vi "Begin.vi"(8 "error in":errorcluster) -> (0 "error out":errorcluster)   [LabVIEW 2014]
doc: "Called before other user functions, this VI is expected to open initial I/O refnums, load in file data, and do all program initialization. Notice that the <B>error out</B> terminal is simply used for data flow. Wiring it to other structures or subVIs ensures that this VI runs first."
uses:
  <vilib>/Rock Robotics/WPI/DriverStation/WPI_DriverStationRobotMode2.ctl
  <vilib>/Rock Robotics/WPI/Joystick/WPI_JoystickDeviceEnum.ctl
  <vilib>/Rock Robotics/SystemInterfaces/DIO/FPGA_DIOChannel.ctl
  <vilib>/Rock Robotics/SystemInterfaces/spilib/spi_bus.ctl
  <vilib>/Rock Robotics/WPI/SafetyOutput/WPI_SafetyOutputConfigMenu.ctl
  <vilib>/Rock Robotics/SystemInterfaces/DIO/FPGA_DIOPWMChannel.ctl
  <vilib>/Rock Robotics/SystemInterfaces/DIO/FPGA_DIORelayChannel.ctl
  <vilib>/Rock Robotics/WPI/Relay/WPI_RelayValue.ctl
  <vilib>/Rock Robotics/SystemInterfaces/i2clib/i2c_bus.ctl
  Robot Global Data.vi
  <vilib>/Rock Robotics/WPI/Counter/WPI_CounterDigitalInputToDigitalSource.vi
  <vilib>/Rock Robotics/WPI/Switch/WPI_SwitchOpenLimit.vi
  <vilib>/Rock Robotics/WPI/RobotDrive/WPI_RobotDriveOpen4MotorWithTalon.vi
  <vilib>/Rock Robotics/WPI/RobotDrive/WPI_RobotDriveOpen4MotorWithCANTalonSRX.vi
  <vilib>/Rock Robotics/WPI/MotorControl/WPI_MotorControlOpen Talon.vi
  SimpleGyro/SimpleGyro.lvlib
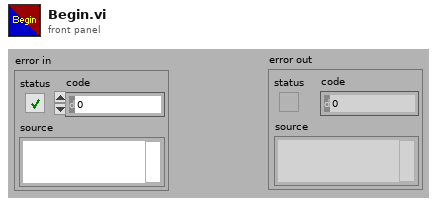
[diagram p1: front panel]
types:
  T1 = typedef "spi_bus.ctl" = enum16{"SPI On-Board, CS0", "SPI On-Board, CS1", "SPI On-Board, CS2", "SPI On-Board, CS3", "SPI MXP", "Invalid"}
  T2 = typedef "FPGA_DIOChannel.ctl" = enum8{"DIO 0", "DIO 1", "DIO 2", "DIO 3", "DIO 4", "DIO 5", "DIO 6", "DIO 7", "DIO 8", "DIO 9", "DIO MXP 0", "DIO MXP 1", "DIO MXP 2", "DIO MXP 3", "DIO MXP 4", "DIO MXP 5", "DIO MXP 6", "DIO MXP 7", "DIO MXP 8", "DIO MXP 9", "DIO MXP 10", "DIO MXP 11", "DIO MXP 12", "DIO MXP 13", "DIO MXP 14", "DIO MXP 15", "Invalid"}
  T3 = typedef "WPI_JoystickDeviceEnum.ctl" = enum16{"USB 0", "USB 1", "USB 2", "USB 3", "USB 4", "USB 5"}
  T4 = typedef "WPI_DriverStationRobotMode2.ctl" = enum16{"Autonomous Disabled", "Autonomous Enabled", "Teleop Disabled", "Teleop Enabled", "Disconnected", "Finish", "Test Disabled", "Test Enabled", "Emergency Stopped"}
  T5 = typedef "WPI_SafetyOutputConfigMenu.ctl" = enum16{"Enable", "Disable"}
  T6 = typedef "FPGA_DIORelayChannel.ctl" = enum8{"Relay 0", "Relay 1", "Relay 2", "Relay 3", "Invalid"}
  T7 = typedef "FPGA_DIOPWMChannel.ctl" = enum8{"PWM 0", "PWM 1", "PWM 2", "PWM 3", "PWM 4", "PWM 5", "PWM 6", "PWM 7", "PWM 8", "PWM 9", "PWM MXP 0", "PWM MXP 1", "PWM MXP 2", "PWM MXP 3", "PWM MXP 4", "PWM MXP 5", "PWM MXP 6", "PWM MXP 7", "PWM MXP 8", "PWM MXP 9", "Invalid"}
  T8 = typedef "WPI_RobotDriveDevRef.ctl" = cluster{"DevStatus":errorcluster, "Motors[]":T9[], "Square Inputs":bool, "Max Output":dbl}
  T9 = typedef "WPI_MotorControlDeviceRef.ctl" = cluster{"DeviceStatus":errorcluster, "Type":T10, "PWM":cluster{"Controller":T11, "PWM Channel":T7, "DeadBand":T12}, "CAN":cluster{"Device Number":u8, "Control Mode":T13, "Semaphore":T14, "Max Vout":dbl, "TalonSRX Control Mode":T15}, "Invert":bool, "TransformRef":T16, "InvTransformRef":T16}
  T10 = typedef "WPI_MotorControlType.ctl" = enum16{"PWM", "CAN", "CANTalonSRX"}
  T11 = typedef "FPGA_TypedefDigitalModule.ctl" = enum16{"Controller 1"}
  T12 = typedef "WPI_PWMDeadband.ctl" = cluster{"Name":string, "maxPositivePwm":i32, "minPositivePwm":i32, "centerPwm":i32, "maxNegativePwm":i32, "minNegativePwm":i32, "angularRange":u16}
  T13 = typedef "WPI_CANJaguar_ControlMode.ctl" = enum8{"Percent VBus", "Current", "Speed", "Position", "Voltage"}
  T14 = typedef "Semaphore RefNum" = refnum<k1>
  T15 = typedef "WPI_CANTalonSRX_APIControlMode.ctl" = enum8{"Percent VBus", "Speed", "Position", "Slave", "Unchanged / Invalid"}
  T16 = typedef "WPI_PWMTransform_ConPane.ctl" = refnum<vi>
  T17 = typedef "WPI_DigitalInputDevRef.ctl" = cluster{"DevStatus":errorcluster, "DIO Channel":T2, "Controller":T11}
  T18 = typedef "FPGA_CounterEncoderSourceConvertionLVSourceType.ctl" = cluster{"DevStatus":errorcluster, "AnalogTriggerMode?":bool, "DigitalMode":cluster{"Controller":T11, "DIO Channel":T19}, "AnalogTriggerMode":cluster{"AnalogTriggerIndex":T20, "OutputType":T21}}
  T19 = typedef "FPGA_DIODigitalSourceChannel.ctl" = enum8{"DIO 0", "DIO 1", "DIO 2", "DIO 3", "DIO 4", "DIO 5", "DIO 6", "DIO 7", "DIO 8", "DIO 9", "DIO MXP 0", "DIO MXP 1", "DIO MXP 2", "DIO MXP 3", "DIO MXP 4", "DIO MXP 5", "DIO MXP 6", "DIO MXP 7", "DIO MXP 8", "DIO MXP 9", "DIO MXP 10", "DIO MXP 11", "DIO MXP 12", "DIO MXP 13", "DIO MXP 14", "DIO MXP 15", "Disabled"}
  T20 = typedef "FPGA_AnalogTriggerIndex.ctl" = enum8{"Trig 0", "Trig 1", "Trig 2", "Trig 3", "Trig 4", "Trig 5", "Trig 6", "Trig 7", "Invalid"}
  T21 = typedef "FPGA_AnalogTriggerOutType.ctl" = enum16{"InWindow", "TriggerState", "Rising", "Falling"}
  T22 = typedef "WPI_EncoderDevRef.ctl" = cluster{"DevStatus":errorcluster, "EncoderIndex":T23, "CounterIndex":T24, "DistancePerCount":dbl, "Decoding Type":T25}
  T23 = typedef "FPGA_EncoderIdx.ctl" = enum8{"Enc 0", "Enc 1", "Enc 2", "Enc 3", "Enc 4", "Enc 5", "Enc 6", "Enc 7", "Invalid"}
  T24 = typedef "FPGA_CounterCtrSystemIndex.ctl" = enum8{"Ctr 0", "Ctr 1", "Ctr 2", "Ctr 3", "Ctr 4", "Ctr 5", "Ctr 6", "Ctr 7", "Invalid"}
  T25 = typedef "WPI_EncoderType.ctl" = enum16{"1x", "2x", "4x"}
  T26 = typedef "WPI_JoystickDevRef.ctl" = cluster{"Device":T3}
  T27 = typedef "SimpleGyro.lvlib/WPI_SimpleGyroDevRef.ctl" = cluster{"DevStatus":errorcluster, "Handle":i32, "Controller":T11, "SPI Bus":T1, "Device Found":bool, "Sample Rate":dbl}
  T28 = typedef "WPI_SwitchDevRef.ctl" = cluster{"DevStatus":errorcluster, "DIO Channel":T2, "Controller":T11, "CntIndex":T24, "Normally Closed":bool}
  T29 = typedef "i2c_bus.ctl" = enum16{"I2C On-Board", "I2C MXP", "Invalid"}
  T30 = typedef "WPI_RelayValue.ctl" = enum16{"Off", "On", "Forward", "Reverse"}
  T31 = typedef "WPI_RelayDevRef.ctl" = cluster{"DevStatus":errorcluster, "Relay Channel":T6, "Controller":T11, "Relay Direction":T32}
  T32 = typedef "WPI_RelayDirection.ctl" = enum16{"Both directions", "Forward only", "Reverse only"}
  T33 = typedef "WPI_I2CDevRef.ctl" = cluster{"DevStatus":errorcluster, "Controller":T11, "Device Address":u8, "Handle":i32, "I2C Bus":T29}
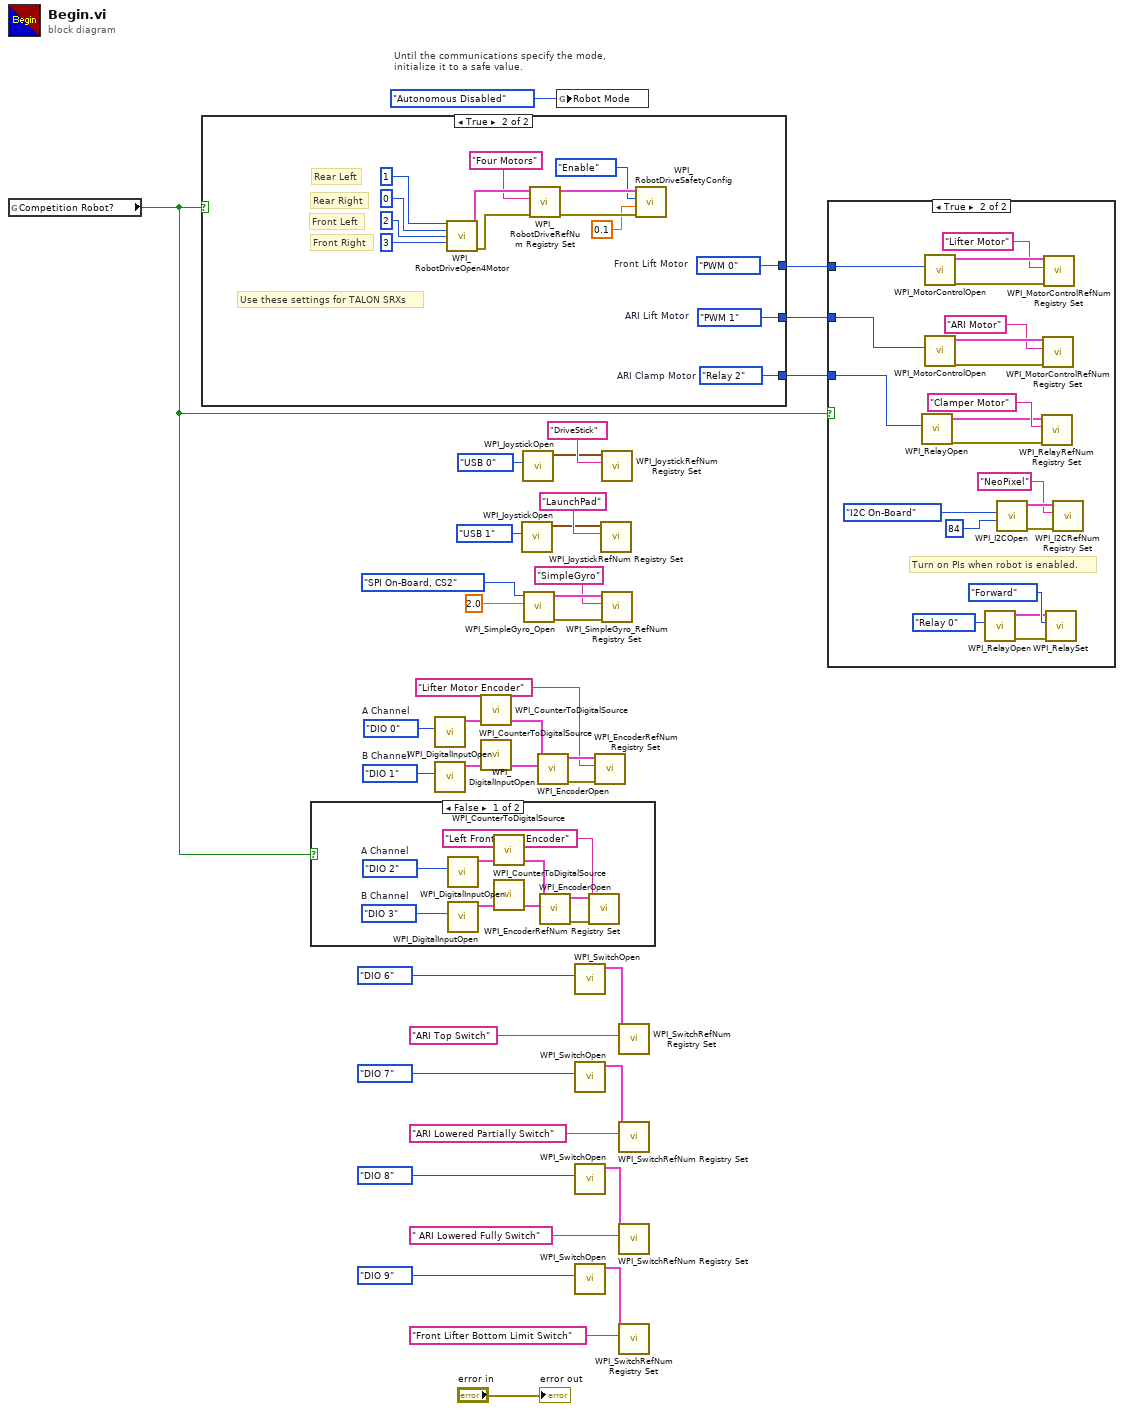
[diagram p0: block diagram]
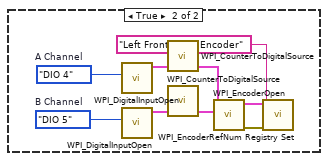
[diagram p2: hidden frame]
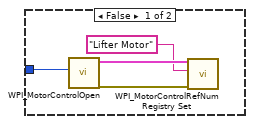
[diagram p3: hidden frame]
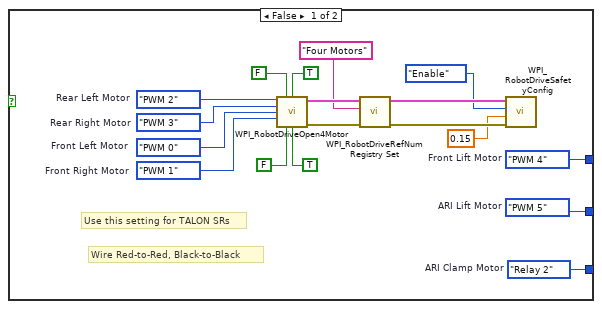
[diagram p4: hidden frame]
diagram:
  w30 = FPGA_DIOChannel."DIO 1"  # B Channel
  w29 = FPGA_DIOChannel."DIO 0"  # A Channel
  # "Until the communications specify the mode,\ninitialize it to a safe value."
  n1 = global read "Robot Global Data.vi" "Competition Robot?"() -> (w1:bool)
  n2 = case shown="True" w1 {
    tunnel: [w47 w61] -> w18
    tunnel: [w46 w60] -> w17
    tunnel: [w45 w59] -> w7
    frame False {
      w45 = FPGA_DIORelayChannel."Relay 2"  # ARI Clamp Motor
      w46 = FPGA_DIOPWMChannel."PWM 5"  # ARI Lift Motor
      w47 = FPGA_DIOPWMChannel."PWM 4"  # Front Lift Motor
      w48 = FPGA_DIOPWMChannel."PWM 1"  # Front Right Motor
      w49 = FPGA_DIOPWMChannel."PWM 0"  # Front Left Motor
      w50 = FPGA_DIOPWMChannel."PWM 3"  # Rear Right Motor
      w51 = FPGA_DIOPWMChannel."PWM 2"  # Rear Left Motor
      # "Wire Red-to-Red, Black-to-Black"
      # "Use this setting for TALON SRs"
      n3 = call-poly <vilib>:"WPI_RobotDriveOpen4Motor.vi"("Rear Left Motor"=w51, "Rear Left Motor Inverted"=FALSE, "Rear Right Motor Inverted"=TRUE, "Rear Right Motor"=w50, "Front Left Motor"=w49, "Front Right Motor"=w48, "Front Left Motor Inverted"=FALSE, "Front Right Motor Inverted"=TRUE) -> ("RobotDriveDevRef"=w56:T8, "error out"=w54:errorcluster)  [unwired: 6 in]
      n4 = call <vilib>:"WPI_RobotDriveRefNum Registry Set.vi"("error in (no error)"=w54, "refnum name"="Four Motors", "RobotDriveDevRef"=w56) -> ("error out"=w40:errorcluster, "RobotDriveDevRef"=w53:T8)  [unwired: 7 out]
      n5 = call <vilib>:"WPI_RobotDriveSafetyConfig.vi"("error in (no error)"=w40, "timeout (s)"=0.15, "mode"=WPI_SafetyOutputConfigMenu."Enable", "RobotDriveDevRef"=w53) -> ()  [unwired: 6 in, 2 out]
    }
    frame True {
      w59 = FPGA_DIORelayChannel."Relay 2"  # ARI Clamp Motor
      w60 = FPGA_DIOPWMChannel."PWM 1"  # ARI Lift Motor
      w61 = FPGA_DIOPWMChannel."PWM 0"  # Front Lift Motor
      # "Use these settings for TALON SRXs"
      # "Front Right"
      # "Front Left"
      # "Rear Right"
      # "Rear Left"
      n6 = call-poly <vilib>:"WPI_RobotDriveOpen4Motor.vi"("Rear Left Motor"=u8 1, "Rear Right Motor"=u8 0, "Front Left Motor"=u8 2, "Front Right Motor"=u8 3) -> ("RobotDriveDevRef"=w70:T8, "error out"=w68:errorcluster)  [unwired: 10 in]
      n7 = call <vilib>:"WPI_RobotDriveRefNum Registry Set.vi"("error in (no error)"=w68, "refnum name"="Four Motors", "RobotDriveDevRef"=w70) -> ("error out"=w58:errorcluster, "RobotDriveDevRef"=w67:T8)  [unwired: 7 out]
      n8 = call <vilib>:"WPI_RobotDriveSafetyConfig.vi"("error in (no error)"=w58, "timeout (s)"=0.1, "mode"=WPI_SafetyOutputConfigMenu."Enable", "RobotDriveDevRef"=w67) -> ()  [unwired: 6 in, 2 out]
    }
  }
  n9 = case shown="False" w1 {
    frame False {
      w79 = FPGA_DIOChannel."DIO 3"  # B Channel
      w78 = FPGA_DIOChannel."DIO 2"  # A Channel
      n10 = call <vilib>:"WPI_DigitalInputOpen.vi"("DIO Channel"=w78) -> ("DigitalInputDevRef"=w75:T17)  [unwired: 2 in, 8 out]
      n11 = call <vilib>:"WPI_DigitalInputOpen.vi"("DIO Channel"=w79) -> ("DigitalInputDevRef"=w76:T17)  [unwired: 2 in, 8 out]
      n12 = call-poly <vilib>:"WPI_CounterToDigitalSource.vi"("DigitalInputDevRef"=w75) -> ("Digital Source"=w74:T18)  [unwired: 6 out]
      n13 = call-poly <vilib>:"WPI_CounterToDigitalSource.vi"("DigitalInputDevRef"=w76) -> ("Digital Source"=w77:T18)  [unwired: 6 out]
      n14 = call <vilib>:"WPI_EncoderOpen.vi"("BSource"=w77, "ASource"=w74) -> ("error out"=w73:errorcluster, "EncoderDevRef"=w72:T22)  [unwired: 6 in, 2 out]
      n15 = call <vilib>:"WPI_EncoderRefNum Registry Set.vi"("error in (no error)"=w73, "refnum name"="Left Front Drive Encoder", "EncoderDevRef"=w72) -> ()  [unwired: 7 in, 2 out]
    }
    frame True {
      w88 = FPGA_DIOChannel."DIO 5"  # B Channel
      w87 = FPGA_DIOChannel."DIO 4"  # A Channel
      n16 = call <vilib>:"WPI_DigitalInputOpen.vi"("DIO Channel"=w87) -> ("DigitalInputDevRef"=w84:T17)  [unwired: 2 in, 8 out]
      n17 = call <vilib>:"WPI_DigitalInputOpen.vi"("DIO Channel"=w88) -> ("DigitalInputDevRef"=w85:T17)  [unwired: 2 in, 8 out]
      n18 = call-poly <vilib>:"WPI_CounterToDigitalSource.vi"("DigitalInputDevRef"=w84) -> ("Digital Source"=w83:T18)  [unwired: 6 out]
      n19 = call-poly <vilib>:"WPI_CounterToDigitalSource.vi"("DigitalInputDevRef"=w85) -> ("Digital Source"=w86:T18)  [unwired: 6 out]
      n20 = call <vilib>:"WPI_EncoderOpen.vi"("BSource"=w86, "ASource"=w83) -> ("error out"=w82:errorcluster, "EncoderDevRef"=w81:T22)  [unwired: 6 in, 2 out]
      n21 = call <vilib>:"WPI_EncoderRefNum Registry Set.vi"("error in (no error)"=w82, "refnum name"="Left Front Drive Encoder", "EncoderDevRef"=w81) -> ()  [unwired: 7 in, 2 out]
    }
  }
  n22 = call <vilib>:"WPI_DigitalInputOpen.vi"("DIO Channel"=w29) -> ("DigitalInputDevRef"=w26:T17)  [unwired: 2 in, 8 out]
  n23 = call <vilib>:"WPI_DigitalInputOpen.vi"("DIO Channel"=w30) -> ("DigitalInputDevRef"=w27:T17)  [unwired: 2 in, 8 out]
  n24 = call-poly <vilib>:"WPI_CounterToDigitalSource.vi"("DigitalInputDevRef"=w26) -> ("Digital Source"=w25:T18)  [unwired: 6 out]
  n25 = call-poly <vilib>:"WPI_CounterToDigitalSource.vi"("DigitalInputDevRef"=w27) -> ("Digital Source"=w28:T18)  [unwired: 6 out]
  n26 = call <vilib>:"WPI_JoystickOpen.vi"("JoystickDevice"=WPI_JoystickDeviceEnum."USB 1") -> ("JoystickDevRef"=w32:T26)  [unwired: 10 in]
  n27 = call <vilib>:"WPI_JoystickOpen.vi"("JoystickDevice"=WPI_JoystickDeviceEnum."USB 0") -> ("JoystickDevRef"=w36:T26)  [unwired: 10 in]
  n28 = call "WPI_SimpleGyro_Open.vi"("Sample Rate (ms)"=2.0, "SPI Chip Select"=spi_bus."SPI On-Board, CS2") -> ("error out"=w5:errorcluster, "SimpleGyroDevRef"=w6:T27)  [unwired: 8 in]
  n29 = call <vilib>:"WPI_EncoderOpen.vi"("BSource"=w28, "ASource"=w25) -> ("error out"=w24:errorcluster, "EncoderDevRef"=w23:T22)  [unwired: 6 in, 2 out]
  n30 = global write "Robot Global Data.vi" "Robot Mode"(WPI_DriverStationRobotMode2."Autonomous Disabled" ("Robot Mode")) -> ()
  n31 = call-poly <vilib>:"WPI_SwitchOpen.vi"("DIO Channel"=FPGA_DIOChannel."DIO 6") -> ("SwitchDevRef"=w14:T28)  [unwired: 9 in, 1 out]
  n32 = call-poly <vilib>:"WPI_SwitchOpen.vi"("DIO Channel"=FPGA_DIOChannel."DIO 7") -> ("SwitchDevRef"=w13:T28)  [unwired: 9 in, 1 out]
  n33 = call-poly <vilib>:"WPI_SwitchOpen.vi"("DIO Channel"=FPGA_DIOChannel."DIO 8") -> ("SwitchDevRef"=w9:T28)  [unwired: 9 in, 1 out]
  n34 = call-poly <vilib>:"WPI_SwitchOpen.vi"("DIO Channel"=FPGA_DIOChannel."DIO 9") -> ("SwitchDevRef"=w20:T28)  [unwired: 9 in, 1 out]
  n35 = call <vilib>:"WPI_EncoderRefNum Registry Set.vi"("error in (no error)"=w24, "refnum name"="Lifter Motor Encoder", "EncoderDevRef"=w23) -> ()  [unwired: 7 in, 2 out]
  n36 = call <vilib>:"WPI_JoystickRefNum Registry Set.vi"("refnum name"="LaunchPad", "JoystickDevRef"=w32) -> ()  [unwired: 8 in, 2 out]
  n37 = call <vilib>:"WPI_JoystickRefNum Registry Set.vi"("refnum name"="DriveStick", "JoystickDevRef"=w36) -> ()  [unwired: 8 in, 2 out]
  n38 = call "WPI_SimpleGyro_RefNum Registry Set.vi"("error in (no error)"=w5, "refnum name"="SimpleGyro", "SimpleGyroDevRef"=w6) -> ()  [unwired: 7 in, 2 out]
  n39 = call <vilib>:"WPI_SwitchRefNum Registry Set.vi"("refnum name"="ARI Top Switch", "SwitchDevRef"=w14) -> ()  [unwired: 8 in, 2 out]
  n40 = call <vilib>:"WPI_SwitchRefNum Registry Set.vi"("refnum name"="ARI Lowered Partially Switch", "SwitchDevRef"=w13) -> ()  [unwired: 8 in, 2 out]
  n41 = call <vilib>:"WPI_SwitchRefNum Registry Set.vi"("refnum name"=" ARI Lowered Fully Switch", "SwitchDevRef"=w9) -> ()  [unwired: 8 in, 2 out]
  n42 = call <vilib>:"WPI_SwitchRefNum Registry Set.vi"("refnum name"="Front Lifter Bottom Limit Switch", "SwitchDevRef"=w20) -> ()  [unwired: 8 in, 2 out]
  n43 = case shown="True" w1 {
    tunnel: w18 -> [w89 w113]
    tunnel: w17 -> [_ w112]
    tunnel: w7 -> [_ w111]
    frame False {
      n44 = call-poly <vilib>:"WPI_MotorControlOpen.vi"("PWM Channel"=w89) -> ("error out"=w91:errorcluster, "MotorControlDeviceRef"=w92:T9)  [unwired: 9 in]
      n45 = call <vilib>:"WPI_MotorControlRefNum Registry Set.vi"("error in (no error)"=w91, "refnum name"="Lifter Motor", "MotorControlDevRef"=w92) -> ()  [unwired: 7 in, 2 out]
    }
    frame True {
      # "Turn on PIs when robot is enabled."
      n46 = call <vilib>:"WPI_RelayOpen.vi"("Relay Channel"=w111) -> ("error out"=w102:errorcluster, "RelayDevRef"=w103:T31)  [unwired: 9 in]
      n47 = call-poly <vilib>:"WPI_MotorControlOpen.vi"("PWM Channel"=w113) -> ("error out"=w109:errorcluster, "MotorControlDeviceRef"=w110:T9)  [unwired: 9 in]
      n48 = call-poly <vilib>:"WPI_MotorControlOpen.vi"("PWM Channel"=w112) -> ("error out"=w106:errorcluster, "MotorControlDeviceRef"=w107:T9)  [unwired: 9 in]
      n49 = call <vilib>:"WPI_RelayOpen.vi"("Relay Channel"=FPGA_DIORelayChannel."Relay 0") -> ("error out"=w99:errorcluster, "RelayDevRef"=w98:T31)  [unwired: 9 in]
      n50 = call <vilib>:"WPI_I2COpen.vi"("Device Address"=u8 84, "I2C Bus"=i2c_bus."I2C On-Board") -> ("error out"=w97:errorcluster, "I2CDevRef"=w96:T33)  [unwired: 8 in]
      n51 = call <vilib>:"WPI_RelayRefNum Registry Set.vi"("error in (no error)"=w102, "refnum name"="Clamper Motor", "RelayDevRef"=w103) -> ()  [unwired: 7 in, 2 out]
      n52 = call <vilib>:"WPI_MotorControlRefNum Registry Set.vi"("error in (no error)"=w106, "refnum name"="ARI Motor", "MotorControlDevRef"=w107) -> ()  [unwired: 7 in, 2 out]
      n53 = call <vilib>:"WPI_MotorControlRefNum Registry Set.vi"("error in (no error)"=w109, "refnum name"="Lifter Motor", "MotorControlDevRef"=w110) -> ()  [unwired: 7 in, 2 out]
      n54 = call <vilib>:"WPI_RelaySet.vi"("error in (no error)"=w99, "RelayValue"=WPI_RelayValue."Forward", "RelayDevRef"=w98) -> ()  [unwired: 7 in, 2 out]
      n55 = call <vilib>:"WPI_I2CRefNum Registry Set.vi"("error in (no error)"=w97, "refnum name"="NeoPixel", "I2CDevRef"=w96) -> ()  [unwired: 7 in, 2 out]
    }
  }
  "error out" <- "error in"
